vi "lockin.GetEvents.RenameMe.vi"(8 "error in (no error)":errorcluster, 11 "system in":refnum<class "system.lvclass">) -> (0 "error out":errorcluster, 3 "System":T3)   [LabVIEW 2016, in "system.lvclass"]
uses:
  system.lvclass
  C:/Program Files (x86)/National Instruments/LabVIEW 2016/vi.lib/JKI/JKI SMO/SMO/SMO.lvclass
  <vilib>/JKI/JKI SMO/SMO/Typedefs/Protected Events.ctl
  <vilib>/JKI/JKI SMO/SMO/Typedefs/StopProcessEventData--Cluster.ctl
  <vilib>/JKI/JKI SMO/SMO/Typedefs/AbortProcessEventData--Cluster.ctl
  <vilib>/JKI/JKI SMO/SMO/Typedefs/SMO Dependency Event--Cluster.ctl
  <vilib>/JKI/JKI SMO/SMO/Typedefs/SMO Dependency Event--Enum.ctl
  Typedefs/PrivateEvents--Cluster.ctl
  Typedefs/PrivateEvents--lockin.output_config.ctl
  Typedefs/PrivateEvents--lockin.runCalculation.ctl
  DSP/Typedefs/LP_Config.ctl
  DSP.lockin/Typedefs/Lockin_Config.ctl
  DSP/Typedefs/FFT_Config.ctl
  <vilib>/Analysis/4window.llb/windowTd.ctl
  <vilib>/measure/maspectr.llb/Power Spectrum and PSD Export Mode.ctl
  Typedefs/PrivateEvents--lockin.lockin_REF_waveform.ctl
  <vilib>/JKI/JKI SMO/SMO/SMO.lvclass
  <vilib>/measure/NI_MAPro.lvlib
  <vilib>/Analysis/NI_AALPro.lvlib
  DSP/DSP.lvclass
  DSP.lockin/DSP_lockin.lvclass
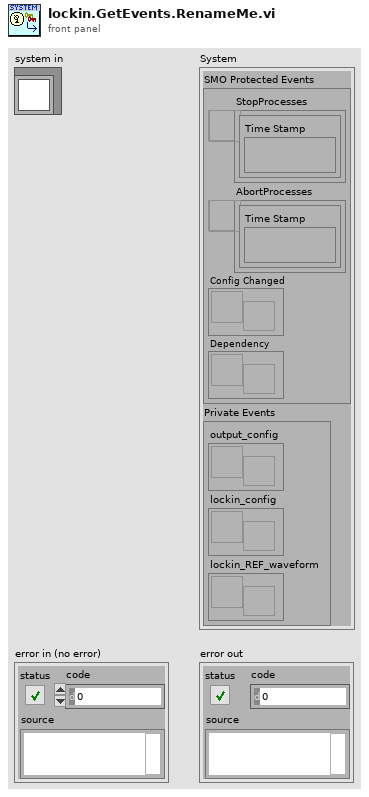
[diagram p1: front panel]
types:
  T1 = typedef "SMO.lvclass/Protected Events.ctl" = cluster{"StopProcesses":refnum<user-event>, "AbortProcesses":refnum<user-event>, "Config Changed":refnum<user-event>, "Dependency":refnum<user-event>}
  T2 = typedef "system.lvclass/PrivateEvents--Cluster.ctl" = cluster{"output_config":refnum<user-event>, "lockin_config":refnum<user-event>, "lockin_REF_waveform":refnum<user-event>}
  T3 = cluster{"SMO Protected Events":T1, "Private Events":T2}
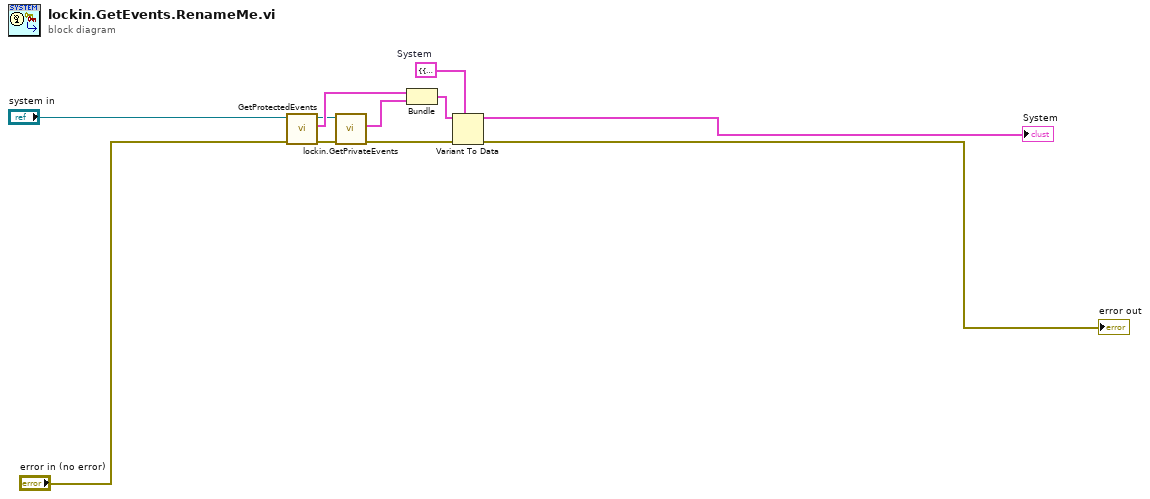
[diagram p0: block diagram]
diagram:
  w6 = T3 {"SMO Protected Events"={"StopProcesses"=refnum, "AbortProcesses"=refnum, "Config Changed"=refnum, "Dependency"=refnum}, "Private Events"={"output_config"=refnum, "lockin_config"=refnum, "lockin_REF_waveform"=refnum}}  # System
  n1 = call <vilib>:"GetProtectedEvents.vi"("error in (no error)"="error in (no error)", "SMO"="system in") -> ("error out"=w5:errorcluster, "SMO Protected Events"=w2:T1, "SMO out"=w1:refnum<class "system.lvclass">)  [unwired: 7 in]
  n2 = call "lockin.GetPrivateEvents.vi"("error in (no error)"=w5, "lockin"=w1) -> ("error out"=w8:errorcluster, "Private Events"=w4:T2)  [unwired: 7 in, 1 out]
  n3 = Bundle("SMO Protected Events"=w2, "Private Events"=w4) -> (w3:T3)  [unwired: 1 in]
  n4 = Variant To Data(error in=w8, type=w6, Variant=w3) -> (data=→"System":T3, error out=→"error out":errorcluster)
